vi "Adding the default value setter Multiple.vi"(0 "VI in":refnum<vi>, 5 "Case Sel Refnum":refnum<vi>, 11 "error in (no error)":errorcluster) -> (4 "VI Out":refnum<vi>, 6 "Case Sel Refnum Out":refnum<vi>, 15 "error out":errorcluster)   [LabVIEW 2021, in "Migrator.lvlib"]
uses:
  Migrator.lvlib
  <vilib>/Utility/miscctls.llb/LVPointTypeDef.ctl
  <vilib>/Utility/miscctls.llb/LVPositionTypeDef.ctl
  Migrator Reusables/Migrator Reusables.lvlib
  Path Functions/Path Functions.lvlib
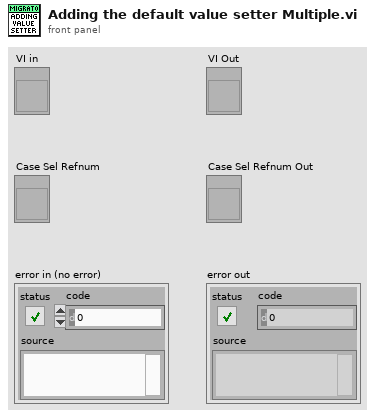
[diagram p1: front panel]
types:
  T1 = typedef "LVPositionTypeDef.ctl" = cluster{"Left":i32, "Top":i32}
  T2 = typedef "LVPointTypeDef.ctl" = cluster{"Horizontal":i16, "Vertical":i16}
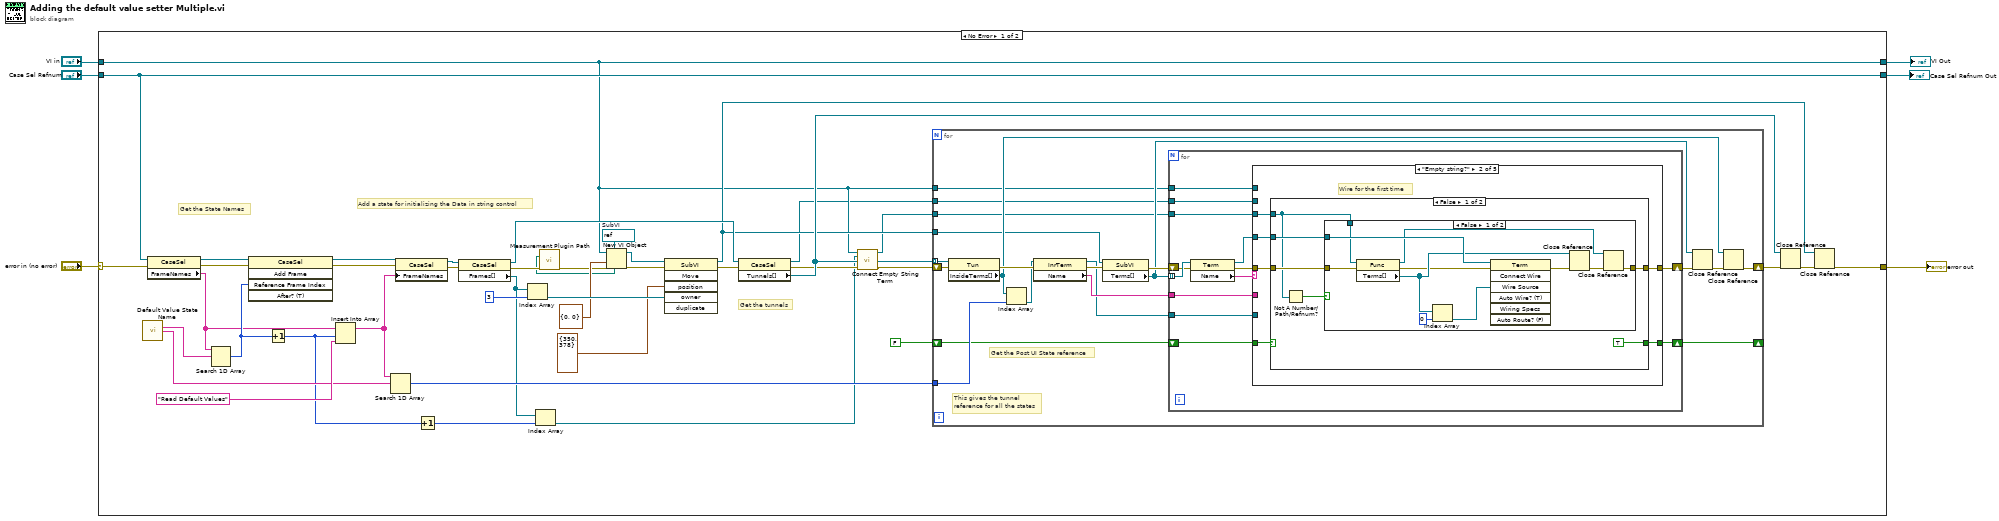
[diagram p0: block diagram]
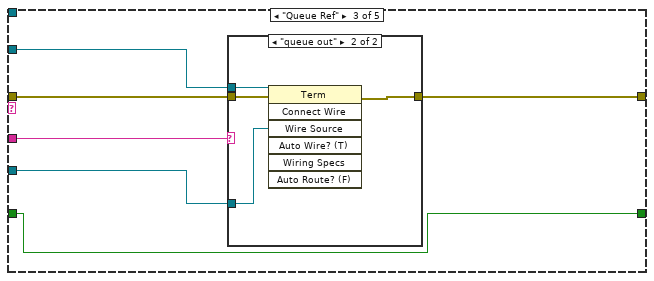
[diagram p5: hidden frame]
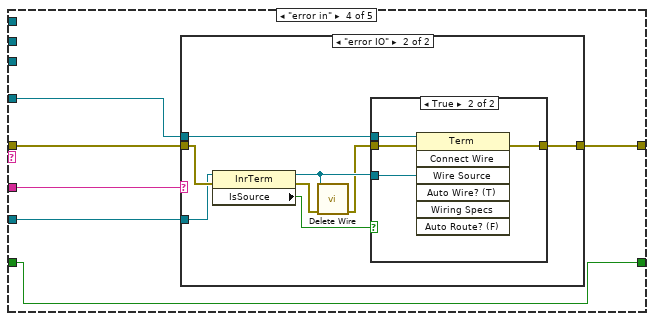
[diagram p7: hidden frame]
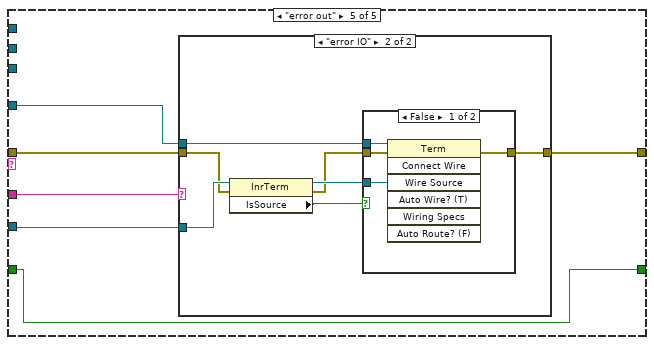
[diagram p10: hidden frame]
diagram:
  n1 = case shown="No Error" "error in (no error)" {
    selector: "error in (no error)" -> [w31 w162]
    tunnel: "Case Sel Refnum" -> [w20 w160]
    tunnel: [w24 w162] -> w5
    tunnel: "VI in" -> [w17 w161]
    tunnel: [w17 w161] -> w2
    tunnel: [w20 w160] -> w1
    frame No Error {
      w33 = refnum<vi> refnum  # SubVI
      # "Get the tunnels"
      # "Add a state for initializing the Data in string control"
      # "Get the State Names"
      n2 = call "Default Value State Name.vi"() -> ("Initialize State"=w22:string, "Post UI Update"=w21:string)  [unwired: 12 in, 2 out]
      n3 = property class="CaseSel"(reference=w20, error in=w31) -> (reference out=w32:refnum<vi>, error out=w30:errorcluster, "FrameNames"=w28:string[])
      n4 = Search 1D Array(1D array=w28, element=w22) -> (index of element=w29:i32)  [unwired: 1 in]
      n5 = invoke class="CaseSel" method="Add Frame"(reference=w32, error in=w30, "Reference Frame Index"=w29) -> (reference out=w38:refnum<vi>, error out=w39:errorcluster)  [unwired: 2 in, 3 out]
      n6 = Increment(x=w29) -> (x+1=w14:i32)
      n7 = Insert Into Array(array=w28, index=w14, new element="Read Default Values" ("new element/subarray")) -> (w47:string[])
      n8 = Search 1D Array(1D array=w47, element=w21) -> (index of element=w48:i32)  [unwired: 1 in]
      n9 = property class="CaseSel"(reference=w38, error in=w39, "FrameNames"=w47) -> (reference out=w42:refnum<vi>, error out=w41:errorcluster)
      n10 = Increment(x=w14) -> (x+1=w11:i32)
      n11 = property class="CaseSel"(reference=w42, error in=w41) -> (reference out=w43:refnum<vi>, error out=w9:errorcluster, "Frames[]"=w15:refnum<vi>[])
      n12 = Index Array(array=w15, index=3) -> (element=w45:refnum<vi>)
      n13 = Index Array(array=w15, index=w11) -> (element=w13:refnum<vi>)
      n14 = call "Measurement Plugin Path.vi"("error in (no error)"=w9) -> ("Set Default Value"=w7:path, "error out"=w8:errorcluster)  [unwired: 2 in, 11 out]
      n15 = New VI Object(vi object class=w33, owner refnum=w17, position/next to=T2 {"Horizontal"=0, "Vertical"=0} ("location"), 6:w7, 8:w8) -> (object refnum=w34:refnum<vi>, 0:w36:errorcluster)  [unwired: 3 in]
      n16 = invoke class="SubVI" method="Move"(reference=w34, error in=w36, "position"=T1 {"Left"=350, "Top"=378}, "owner"=w45) -> (reference out=w23:refnum<vi>, error out=w46:errorcluster)  [unwired: 2 in, 4 out]
      n17 = property class="CaseSel"(reference=w43, error in=w46) -> (reference out=w16:refnum<vi>, error out=w18:errorcluster, "Tunnels[]"=w26:refnum<vi>[])
      n18 = call "Connect Empty String Term.vi"("VI Refnum"=w17, "State Refnum"=w13, "error in (no error)"=w18) -> ("Func Refnum"=w12:refnum<vi>, "error out"=w19:errorcluster)  [unwired: 11 in]
      n19 = for {
        tunnel: w26 -> [w67] mode=indexing
        shift-right: [w59] -> w27
        shift-left: w19 -> [w68]
        tunnel: w48 -> [w66]
        tunnel: w23 -> [w54]
        tunnel: w16 -> [w53]
        tunnel: w17 -> [w52]
        tunnel: w12 -> [w51]
        shift-right: [w49] -> _
        shift-left: FALSE -> [w50]
        # "Get the Post UI State reference"
        # "This gives the tunnel \nreference for all the states"
        n20 = property class="Tun"(reference=w67, error in=w68) -> (error out=w65:errorcluster, "InsideTerms[]"=w58:refnum<vi>[])  [unwired: 1 out]
        n21 = Index Array(array=w58, index=w66) -> (element=w60:refnum<vi>)
        n22 = property class="InrTerm"(reference=w60, error in=w65) -> (reference out=w61:refnum<vi>, error out=w64:errorcluster, "Name"=w62:string)
        n23 = property class="SubVI"(reference=w54, error in=w64) -> (error out=w63:errorcluster, "Terms[]"=w57:refnum<vi>[])  [unwired: 1 out]
        n24 = for {
          tunnel: w57 -> [w81] mode=indexing
          tunnel: w62 -> [w78]
          tunnel: w61 -> [w75]
          shift-right: [w74] -> w55
          shift-left: w63 -> [w80]
          tunnel: w53 -> [w73]
          tunnel: w52 -> [w72]
          tunnel: w51 -> [w71]
          shift-right: [w69] -> w49
          shift-left: w50 -> [w70]
          n25 = property class="Term"(reference=w81, error in=w80) -> (reference out=w77:refnum<vi>, error out=w76:errorcluster, "Name"=w79:string)
          n26 = case shown="\"Empty string?\"" w79 {
            tunnel: w78 -> [_ _ w115 w125 w146]
            tunnel: w77 -> [_ w89 w114 w123 w144]
            tunnel: w76 -> [w83 w87 w113 w126 w145]
            tunnel: w75 -> [_ _ w112 w122 w143]
            tunnel: [w83 w86 w111 w124 w142] -> w74
            tunnel: w73 -> [_ _ _ _ _]
            tunnel: w72 -> [_ _ _ _ _]
            tunnel: w71 -> [_ w88 _ _ _]
            tunnel: w70 -> [w82 w84 w110 w121 w141]
            tunnel: [w82 w85 w110 w121 w141] -> w69
            frame Default {
            }
            frame "Empty string?" {
              # "Wire for the first time"
              n27 = case shown="False" w84 {
                selector: w84 -> [_ w108]
                tunnel: w89 -> [w95 _]
                tunnel: w88 -> [w91 _]
                tunnel: w87 -> [w94 w109]
                tunnel: [w93 w109] -> w86
                tunnel: [TRUE w108] -> w85
                frame False {
                  n28 = Not A Number/Path/Refnum?(number/path/refnum=w91) -> (NaN/Path/Refnum?=w90:bool)
                  n29 = case shown="False" w90 {
                    tunnel: w95 -> [w106 _]
                    tunnel: w94 -> [w100 w107]
                    tunnel: [w98 w107] -> w93
                    tunnel: w91 -> [w96 _]
                    frame False {
                      n30 = property class="Func"(reference=w96, error in=w100) -> (reference out=w97:refnum<vi>, error out=w99:errorcluster, "Terms[]"=w101:refnum<vi>[])
                      n31 = Index Array(array=w101, index=0) -> (element=w104:refnum<vi>)
                      n32 = invoke class="Term" method="Connect Wire"(reference=w106, error in=w99, "Wire Source"=w104) -> (error out=w103:errorcluster)  [unwired: 4 in, 6 out]
                      n33 = Close Reference(reference=w101, error in (no error)=w103) -> (error out=w102:errorcluster)
                      n34 = Close Reference(reference=w97, error in (no error)=w102) -> (error out=w98:errorcluster)
                    }
                    frame True {
                    }
                  }
                }
                frame True {
                }
              }
            }
            frame "Queue Ref" {
              n35 = case shown="\"queue out\"" w115 {
                tunnel: w114 -> [_ w119]
                tunnel: w113 -> [w116 w120]
                tunnel: w112 -> [_ w118]
                tunnel: [w116 w117] -> w111
                frame Default {
                }
                frame "queue out" {
                  n36 = invoke class="Term" method="Connect Wire"(reference=w119, error in=w120, "Wire Source"=w118) -> (error out=w117:errorcluster)  [unwired: 4 in, 6 out]
                }
              }
            }
            frame "error in" {
              n37 = case shown="\"error IO\"" w125 {
                tunnel: w126 -> [w127 w133]
                tunnel: w123 -> [_ w135]
                tunnel: [w127 w134] -> w124
                tunnel: w122 -> [_ w132]
                frame Default {
                }
                frame "error IO" {
                  n38 = property class="InrTerm"(reference=w132, error in=w133) -> (reference out=w130:refnum<vi>, error out=w129:errorcluster, "IsSource"=w131:bool)
                  n39 = call "Delete Wire.vi"("Terminal Reference"=w130, "error in (no error)"=w129) -> ("error out"=w128:errorcluster)  [unwired: 13 in]
                  n40 = case shown="True" w131 {
                    tunnel: w135 -> [_ w140]
                    tunnel: [w136 w139] -> w134
                    tunnel: w130 -> [_ w138]
                    tunnel: w128 -> [w136 w137]
                    frame False {
                    }
                    frame True {
                      n41 = invoke class="Term" method="Connect Wire"(reference=w140, error in=w137, "Wire Source"=w138) -> (error out=w139:errorcluster)  [unwired: 4 in, 6 out]
                    }
                  }
                }
              }
            }
            frame "error out" {
              n42 = case shown="\"error IO\"" w146 {
                tunnel: w145 -> [w147 w150]
                tunnel: w144 -> [_ w154]
                tunnel: w143 -> [_ w152]
                tunnel: [w147 w153] -> w142
                frame Default {
                }
                frame "error IO" {
                  n43 = property class="InrTerm"(reference=w152, error in=w150) -> (reference out=w151:refnum<vi>, error out=w149:errorcluster, "IsSource"=w148:bool)
                  n44 = case shown="False" w148 {
                    tunnel: w154 -> [w158 _]
                    tunnel: [w157 w159] -> w153
                    tunnel: w151 -> [w156 _]
                    tunnel: w149 -> [w155 w159]
                    frame False {
                      n45 = invoke class="Term" method="Connect Wire"(reference=w158, error in=w155, "Wire Source"=w156) -> (error out=w157:errorcluster)  [unwired: 4 in, 6 out]
                    }
                    frame True {
                    }
                  }
                }
              }
            }
          }
        }
        n46 = Close Reference(reference=w57, error in (no error)=w55) -> (error out=w56:errorcluster)
        n47 = Close Reference(reference=w58, error in (no error)=w56) -> (error out=w59:errorcluster)
      }
      n48 = Close Reference(reference=w26, error in (no error)=w27) -> (error out=w25:errorcluster)
      n49 = Close Reference(reference=w23, error in (no error)=w25) -> (error out=w24:errorcluster)
    }
    frame Error {
    }
  }
  "error out" <- w5
  "VI Out" <- w2
  "Case Sel Refnum Out" <- w1
